vi "Update-and-display-processing-stats.vi"(8 "error in":errorcluster, 10 "Data ref. in":refnum<data-value>, 11 "UI ref. in":refnum<data-value>) -> (0 "error IO":errorcluster, 2 "Data ref.":refnum<data-value>, 3 "UI ref.":refnum<data-value>)   [LabVIEW 2013, in "CameraVision.lvlib" / "CV-UI.lvclass"]
uses:
  CV-UI.lvclass
  Main/CV-Main.lvclass
  Display-names.ctl
  Main/CV-Main.lvclass/CV-Main.ctl
  Main/Buffers/CV-Buffers.lvclass/CV-Buffers.ctl
  Main/Read Buffers.vi
  Main/Buffers/Read Processing buffer.vi
  Main/Buffers/Read Storage buffer.vi
  Main/Buffers/CV-Buffers.lvclass
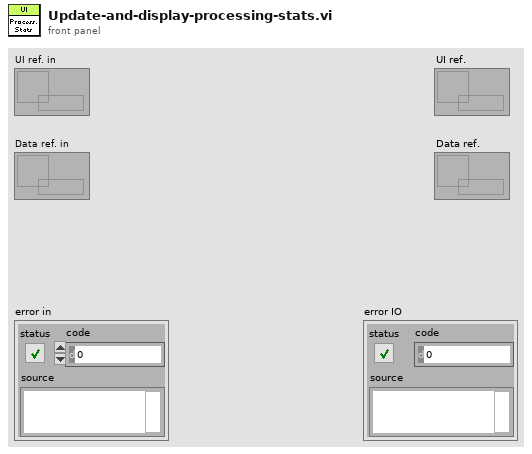
[diagram p1: front panel]
types:
  T1 = typedef "CameraVision.lvlib/CV-UI.lvclass/Display-names.ctl" = enum16{"State", "Action", "Current image", "Framerate", "Frametime", "Process buffer", "Storage buffer", "Free disk space", "Total disk space", "Information", "Histogram", "Camera 1", "Camera 2", "Camera 1 chart", "Camera 2 chart", "Browser", "Temperature", "Map", "Status overview", "Characteristics", "Temper characteristics"}
  T2 = typedef "CameraVision.lvlib/CV-Acquisition.lvclass/Acquisition-stats.ctl" = cluster{"Index":i32, "Time":timestamp, "Acq duration":dbl, "Process duration":dbl}
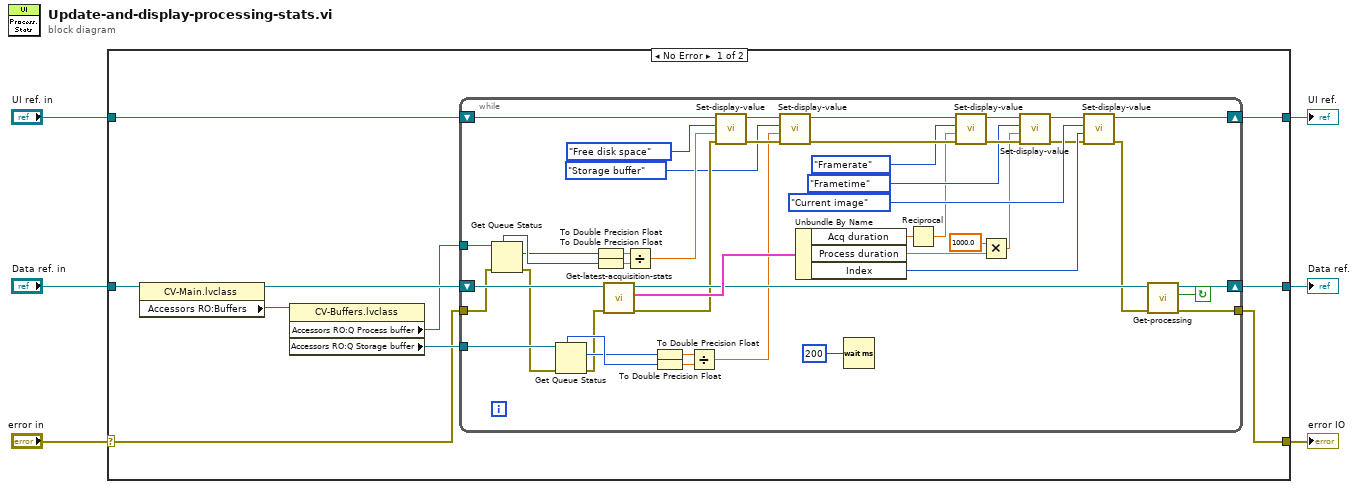
[diagram p0: block diagram]
diagram:
  n1 = case shown="No Error" "error in" {
    selector: "error in" -> [w7 w64]
    tunnel: [w16 w64] -> w6
    tunnel: "UI ref. in" -> [w8 w63]
    tunnel: "Data ref. in" -> [w15 w62]
    tunnel: [w10 w63] -> w2
    tunnel: [w11 w62] -> w1
    frame No Error {
      n2 = property class="CV-Main.lvclass"(reference=w15) -> (reference out=w14:refnum<data-value>, "Accessors RO:Buffers"=w13:refnum<class "CV-Buffers.lvclass">)  [unwired: 1 in, 1 out]
      n3 = property class="CV-Buffers.lvclass"(reference=w13) -> ("Accessors RO:Q Process buffer"=w12:refnum<queue>, "Accessors RO:Q Storage buffer"=w9:refnum<queue>)  [unwired: 1 in, 2 out]
      n4 = while {
        tunnel: [w38] -> w16
        shift-right: [w57] -> w11
        shift-left: w14 -> [w60]
        shift-right: [w41] -> w10
        shift-left: w8 -> [w56]
        tunnel: w12 -> [w54]
        tunnel: w7 -> [w53]
        tunnel: w9 -> [w33]
        stop <- w39 continue-if-true
        (unwired) Display-names."Frametime" ("Display name")
        n5 = Get Queue Status(queue=w54, error in (no error)=w53) -> (max queue size=w52:i32, # pending remove=w51:i32, error out=w32:errorcluster)  [unwired: 1 in, 5 out]
        n6 = Get Queue Status(queue=w33, error in (no error)=w32) -> (max queue size=w37:i32, # pending remove=w36:i32, error out=w31:errorcluster)  [unwired: 1 in, 5 out]
        n7 = To Double Precision Float(number=w51) -> (double precision float=w50:dbl)
        n8 = To Double Precision Float(number=w52) -> (double precision float=w49:dbl)
        n9 = call "Get-latest-acquisition-stats.vi"("error in (no error)"=w31, "Data ref. in"=w60) -> ("error out"=w47:errorcluster, "Acq stats"=w59:T2, "Data ref."=w58:refnum<data-value>)  [unwired: 7 in]
        n10 = Divide(x=w50, y=w49) -> (x/y=w48:dbl)
        n11 = To Double Precision Float(number=w36) -> (double precision float=w35:dbl)
        n12 = To Double Precision Float(number=w37) -> (double precision float=w34:dbl)
        n13 = Divide(x=w35, y=w34) -> (x/y=w27:dbl)
        n14 = call "Set-display-value.vi"("error in (no error)"=w47, "Value"=w48, "Display name"=Display-names."Free disk space", "UI ref. in"=w56) -> ("error out"=w29:errorcluster, "UI ref."=w30:refnum<data-value>)  [unwired: 6 in]
        n15 = call "Set-display-value.vi"("error in (no error)"=w29, "Value"=w27, "Display name"=Display-names."Storage buffer", "UI ref. in"=w30) -> ("error out"=w25:errorcluster, "UI ref."=w26:refnum<data-value>)  [unwired: 6 in]
        n16 = Unbundle By Name(w59) -> ("Acq duration"=w22:dbl, "Process duration"=w46:dbl, "Index"=w43:i32)
        n17 = Wait (ms)(milliseconds to wait=u32 200 ("Update interval (ms)")) -> ()  [unwired: 1 out]
        n18 = Reciprocal(x=w22) -> (1/x=w19:dbl)
        n19 = call "Set-display-value.vi"("error in (no error)"=w25, "Value"=w19, "Display name"=Display-names."Framerate", "UI ref. in"=w26) -> ("error out"=w23:errorcluster, "UI ref."=w24:refnum<data-value>)  [unwired: 6 in]
        n20 = Multiply(x=1000.0 ("y"), y=w46) -> (x*y=w18:dbl)
        n21 = call "Set-display-value.vi"("error in (no error)"=w23, "Value"=w18, "Display name"=Display-names."Frametime", "UI ref. in"=w24) -> ("error out"=w42:errorcluster, "UI ref."=w45:refnum<data-value>)  [unwired: 6 in]
        n22 = call "Set-display-value.vi"("error in (no error)"=w42, "Value"=w43, "Display name"=Display-names."Current image", "UI ref. in"=w45) -> ("error out"=w40:errorcluster, "UI ref."=w41:refnum<data-value>)  [unwired: 6 in]
        n23 = call "Get-processing.vi"("error in (no error)"=w40, "Data ref. in"=w58) -> ("error out"=w38:errorcluster, "Processing?"=w39:bool, "Data ref."=w57:refnum<data-value>)  [unwired: 7 in]
      }
    }
    frame Error {
    }
  }
  "error IO" <- w6
  "Data ref." <- w1
  "UI ref." <- w2
